vi "point(8x).vi"(5 "Frequency":dbl=60.5, 6 "delta f":dbl=0.25000000023283064, 7 "Input VdB":dbl[](array[numeric])=array[8192 elements]) -> (0 "mils/sec":ext=2.3668537178741005 format="%#.3f", 1 "dB (AdB)":dbl=64.16006344482969 format="%#.2f", 2 "dB (VdB)":ext=72.55289843818935 format="%#.2f", 3 "mag. (Vpeak)":dbl=0.02364404242483217)   [LabVIEW 2010]
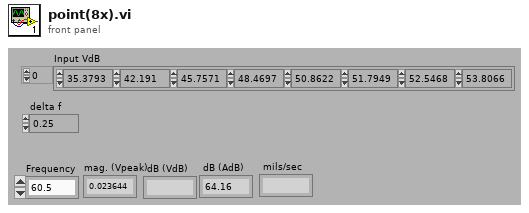
[diagram p1: front panel]
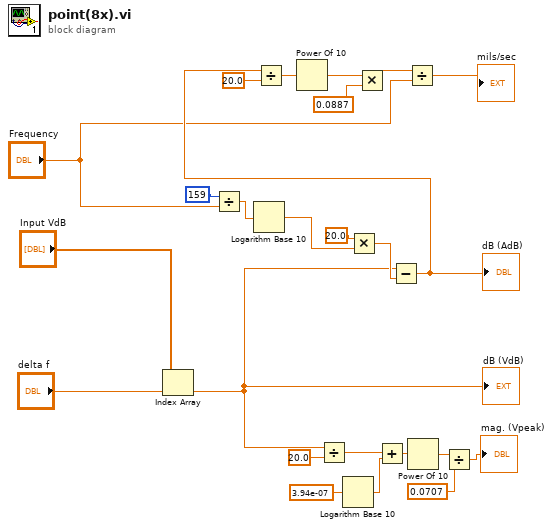
[diagram p0: block diagram]
diagram:
  n1 = Index Array(array="Input VdB", index="delta f") -> (element=w2:dbl)
  "dB (VdB)" <- w2
  n2 = Divide(x=159, y="Frequency") -> (x/y=w18:dbl)
  n3 = Logarithm Base 10(1:w18) -> (0:w17:dbl)
  n4 = Divide(x=w2, y=20.0) -> (x/y=w23:dbl)
  n5 = Logarithm Base 10(1:3.94e-07 ("x")) -> (0:w22:dbl)
  n6 = Multiply(x=20.0, y=w17) -> (x*y=w15:dbl)
  n7 = Add(x=w23, y=w22) -> (x+y=w20:dbl)
  n8 = Subtract(x=w2, y=w15) -> (x-y=w10:dbl)
  "dB (AdB)" <- w10
  n9 = Divide(x=w10, y=20.0) -> (x/y=w8:dbl)
  n10 = Power Of 10(x=w8) -> (10^x=w6:dbl)
  n11 = Multiply(x=w6, y=0.0887) -> (x*y=w5:dbl)
  n12 = Divide(x=w5, y="Frequency") -> (x/y=→"mils/sec":dbl)
  n13 = Power Of 10(x=w20) -> (10^x=w13:dbl)
  n14 = Divide(x=w13, y=0.0707) -> (x/y=→"mag. (Vpeak)":dbl)
